vi "Find Ballard MIL-STD-1553 Custom Device.vi"(8 "error in":errorcluster, 10 "name":string, 11 "target in":refnum<k24>) -> (0 "error out":errorcluster, 2 "Ballard MIL-STD-1553 custom device":u64, 3 "target out":refnum<k24>, 4 "found?":bool)   [LabVIEW 2020, in "Ballard MIL-STD-1553 Scripting.lvlib"]
doc: "Within the specified target, this VI searches for the named Ballard MIL-STD-1553 custom device and returns a reference to the found <b>Ballard MIL-STD-1553 custom device</b>."
uses:
  Ballard MIL-STD-1553 Scripting.lvlib
  NationalInstruments.VeriStand.SystemDefinitionAPI
  Constants.vi
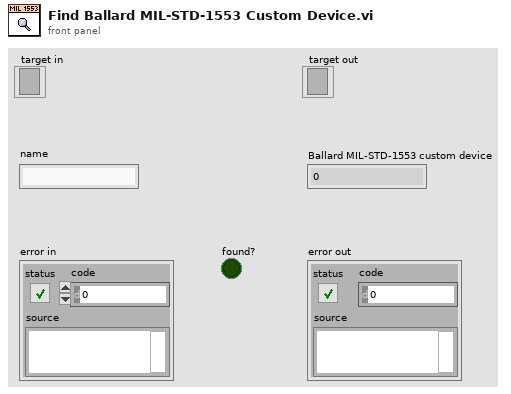
[diagram p1: front panel]
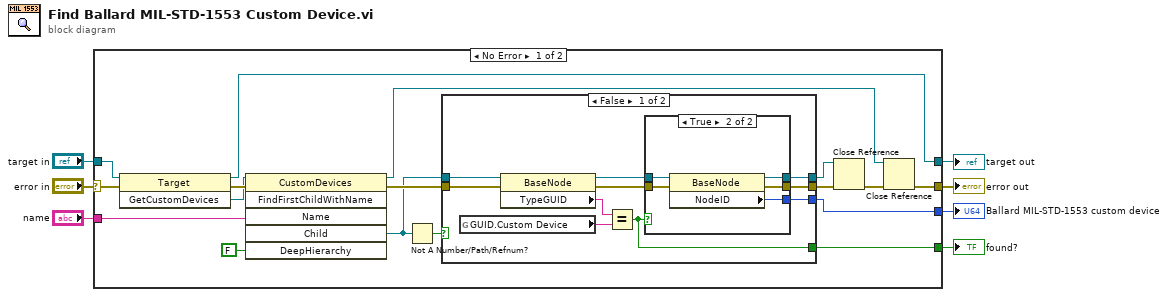
[diagram p0: block diagram]
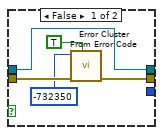
[diagram p2: hidden frame]
diagram:
  n1 = case shown="No Error" "error in" {
    selector: "error in" -> [w19 w48]
    tunnel: "target in" -> [w20 w47]
    tunnel: [w14 w48] -> w5
    tunnel: [w11 _] -> w2
    tunnel: [w16 w47] -> w4
    tunnel: "name" -> [w13 _]
    tunnel: [w8 _] -> w1
    frame No Error {
      n2 = invoke on="Invoke Node" class="Target" method="GetCustomDevices"(reference=w20, error in=w19) -> (reference out=w16:refnum<k24>, error out=w24:errorcluster, "GetCustomDevices"=w23:refnum<k24>)  [unwired: 1 in]
      n3 = invoke on="Invoke Node" class="CustomDevices" method="FindFirstChildWithName"(reference=w23, error in=w24, "Name"=w13, "DeepHierarchy"=FALSE) -> (reference out=w17:refnum<k24>, error out=w15:errorcluster, "Child"=w12:refnum<k24>)  [unwired: 2 in, 3 out]
      n4 = Not A Number/Path/Refnum?(number/path/refnum=w12) -> (NaN/Path/Refnum?=w10:bool)
      n5 = case shown="False" w10 {
        tunnel: [w34 w45] -> w22
        tunnel: [w33 w46] -> w21
        tunnel: w15 -> [w31 w46]
        tunnel: w12 -> [w30 w45]
        tunnel: [w32 _] -> w11
        tunnel: [w25 _] -> w8
        frame False {
          n6 = global read "Constants.vi" "GUID.Custom Device"() -> (w28:string)
          n7 = property on="Property Node" class="BaseNode"(reference=w30, error in=w31) -> (reference out=w26:refnum<k24>, error out=w27:errorcluster, "TypeGUID"=w29:string)
          n8 = Equal?(x=w29, y=w28) -> (x = y?=w25:bool)
          n9 = case shown="True" w25 {
            tunnel: [w36 w41] -> w33
            tunnel: w27 -> [w38 w43]
            tunnel: w26 -> [w39 w44]
            tunnel: [w39 w42] -> w34
            tunnel: [_ w40] -> w32
            frame False {
              n10 = call <vilib>:"Error Cluster From Error Code.vi"("show call chain? (False)"=TRUE, "error in (no error)"=w38, "error code (0)"=-732350) -> ("error out"=w36:errorcluster)  [unwired: 6 in]
            }
            frame True {
              n11 = property on="Property Node" class="BaseNode"(reference=w44, error in=w43) -> (reference out=w42:refnum<k24>, error out=w41:errorcluster, "NodeID"=w40:u64)
            }
          }
        }
        frame True {
        }
      }
      n12 = Close Reference(reference=w22, error in (no error)=w21) -> (error out=w18:errorcluster)
      n13 = Close Reference(reference=w17, error in (no error)=w18) -> (error out=w14:errorcluster)
    }
    frame Error {
    }
  }
  "error out" <- w5
  "target out" <- w4
  "Ballard MIL-STD-1553 custom device" <- w2
  "found?" <- w1
